vi "Read Config.vi"(8 "error in (no error)":errorcluster, 11 "FileName":string="SerialConfig.xml") -> (0 "error out":errorcluster, 3 "Serial Config":T1={"串口选择"="", "通讯速率"=9600, "超时时间"=10000, "数据位长"=8, "奇偶校验"=enum."None", "停止位长"=10, "握手控制"=0, "字符结束"=TRUE, "结束字符"=10, "仪器地址"=1} {"结束字符" format="%.0x"; "握手控制" items=["None", "XON/XOFF", "RTS/CTS", "XON/XOFF & RTS/CTS", "DTR/DSR", "XON/XOFF & DTR/DSR"]; "停止位长" items=["1.0"=10, "1.5"=15, "2.0"=20]; "数据位长" min=5 max=8 step=1})   [LabVIEW 2010, in "CM51.lvlib"]
doc: "Use this template to build a VI to use as a subVI."
uses:
  CM51.lvlib
  Serial Config.ctl
  <vilib>/Utility/xml.llb/Read From XML File(string).vi
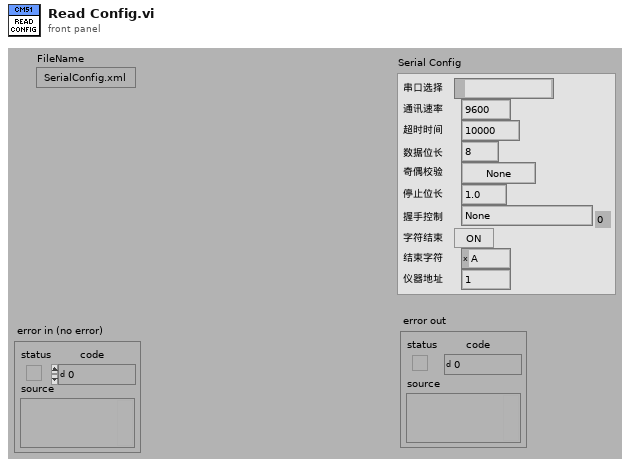
[diagram p1: front panel]
types:
  T1 = typedef "CM51.lvlib/Serial Config.ctl" = cluster{"串口选择":refnum<visa-resource-name>, "通讯速率":u32, "超时时间":u32, "数据位长":u16, "奇偶校验":enum16{"None", "Odd", "Even", "Mark", "Space"}, "停止位长":u16, "握手控制":u16, "字符结束":bool, "结束字符":u8, "仪器地址":u32}
  T2 = enum32{"invalid app kind", "Development System", "Run Time System", "Student Edition", "Embedded LabVIEW", "Evaluation", "Custom"}
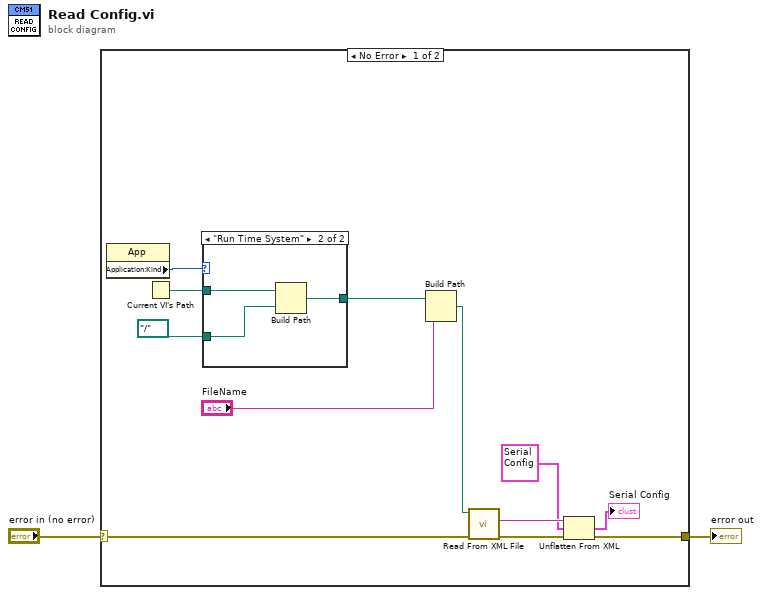
[diagram p0: block diagram]
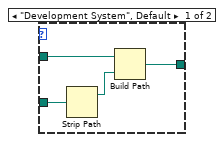
[diagram p2: hidden frame]
diagram:
  n1 = case shown="No Error" "error in (no error)" {
    selector: "error in (no error)" -> [w7 w22]
    tunnel: [w5 w22] -> w1
    frame No Error {
      n2 = property class="App"() -> ("Application:Kind"=w9:T2)  [unwired: 2 in, 2 out]
      n3 = Current VI's Path() -> (path=w10:path)
      n4 = case shown="\"Run Time System\"" w9 {
        tunnel: [w18 w19] -> w12
        tunnel: w10 -> [w17 w21]
        tunnel: path "../.." ("relative path (.)") -> [w16 w20]
        frame "Development System", Default {
          n5 = Strip Path(path=w16) -> (stripped path=w15:path)  [unwired: 1 out]
          n6 = Build Path(base path=w17, name or relative path=w15) -> (appended path=w18:path)
        }
        frame "Run Time System" {
          n7 = Build Path(base path=w21, name or relative path=w20) -> (appended path=w19:path)
        }
      }
      n8 = Build Path(base path=w12, name or relative path="FileName") -> (appended path=w14:path)
      n9 = call-poly <vilib>:"Read From XML File.vi"("error in (no error)"=w7, "XML File Path"=w14) -> ("error out"=w6:errorcluster, "XML Elements"=w8:string)  [unwired: 7 in, 1 out]
      n10 = Unflatten From XML(xml string=w8, type=T1 {"串口选择"="", "通讯速率"=9600, "超时时间"=10000, "数据位长"=8, "奇偶校验"=enum."None", "停止位长"=10, "握手控制"=0, "字符结束"=TRUE, "结束字符"=10, "仪器地址"=1} ("Serial Config 2"), error in (no error)=w6) -> (value=→"Serial Config":T1, error out=w5:errorcluster)
    }
    frame Error {
    }
  }
  "error out" <- w1
